vi "SoundCard-Write Data to Stream.vi"(0 "task ID":T1 format="%.0x", 7 "Array":dbl[](array[numeric]), 11 "error in (no error)":errorcluster) -> (4 "task ID out":T1 format="%.0x", 15 "error out":errorcluster)   [LabVIEW 2020]
uses:
  <vilib>/sound2/lvsound2.llb/Sound Output Task ID.ctl
  <vilib>/sound2/lvsound2.llb/Sound Output Write (DBL).vi
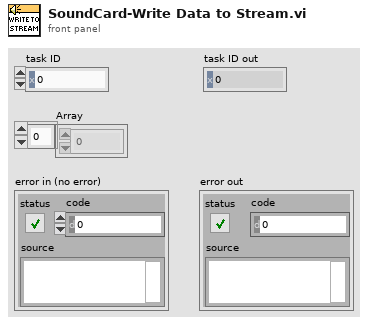
[diagram p1: front panel]
types:
  T1 = typedef "Sound Output Task ID.ctl" = u32
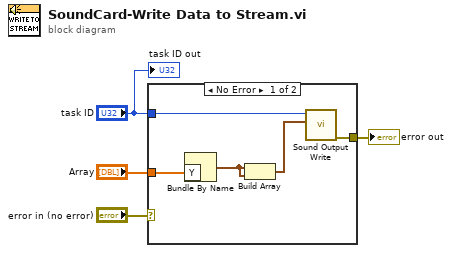
[diagram p0: block diagram]
diagram:
  n1 = case shown="No Error" "error in (no error)" {
    selector: "error in (no error)" -> [_ w10]
    tunnel: [w5 w10] -> w2
    tunnel: "Array" -> [w7 _]
    tunnel: "task ID" -> [w6 _]
    frame No Error {
      n2 = Bundle By Name("Y"=w7) -> (w8:waveform(dbl))  [unwired: 1 in]
      n3 = Build Array(w8, w8) -> (w9:waveform(dbl)[])
      n4 = call-poly <vilib>:"Sound Output Write.vi"("data"=w9, "task ID"=w6) -> ("error out"=w5:errorcluster)  [unwired: 8 in, 1 out]
    }
    frame Error {
    }
  }
  "error out" <- w2
  "task ID out" <- "task ID"
